vi "Uniform (Discrete) Inverse CDF.vi"(10 "n":i32=100, 11 "cdf(x)":dbl) -> (0 "error":i32, 3 "x":i32)   [LabVIEW 2017, in "NI_Gmath.lvlib"]
doc: "Computes the discrete inverse cumulative distribution function (CDF), or the value <B>x</B> such that the probability that the random variate X, where X describes the selected distribution type, takes on a value less than or equal to it is <B>cdf(x)</B>. You must manually select the polymorphic instance to use."
uses:
  NI_Gmath.lvlib
  st_error_code.ctl
panel:
  # "Uniform (Discrete) Inverse CDF"
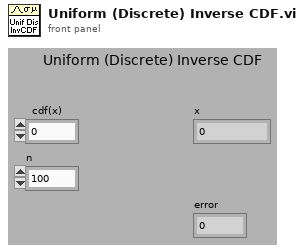
[diagram p1: front panel]
types:
  T1 = typedef "NI_Gmath.lvlib/st_error_code.ctl" = i32
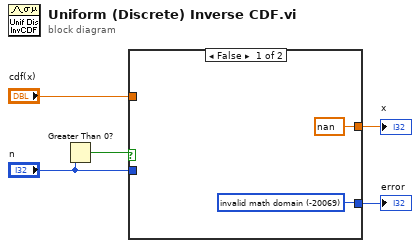
[diagram p0: block diagram]
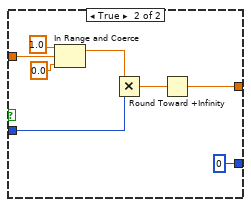
[diagram p2: hidden frame]
diagram:
  n1 = Greater Than 0?(x="n") -> (x > 0?=w3:bool)
  n2 = case shown="False" w3 {
    tunnel: [nan w8] -> w5
    tunnel: [w6 0 ("invalid math domain")] -> w4
    tunnel: "cdf(x)" -> [_ w14]
    tunnel: "n" -> [_ w10]
    frame False {
      w6 = T1 -20069 items=["invalid math domain"=-20069, "Fourier interpolation size m >= n"=-20070, "empty array"=-20003] ("stat interp error code")
    }
    frame True {
      n3 = In Range and Coerce(upper limit=1.0 ("lower limit"), x=w14, lower limit=0.0) -> (coerced(x)=w11:dbl)  [unwired: 1 out]
      n4 = Multiply(x=w11, y=w10) -> (x*y=w9:dbl)
      n5 = Round Toward +Infinity(x=w9) -> (ceil(x): smallest int >= x=w8:dbl)
    }
  }
  "x" <- w5
  "error" <- w4
